vi "Delete remainig  reports at the begining.vi"() -> (0 "error out":errorcluster)   [LabVIEW 2023]
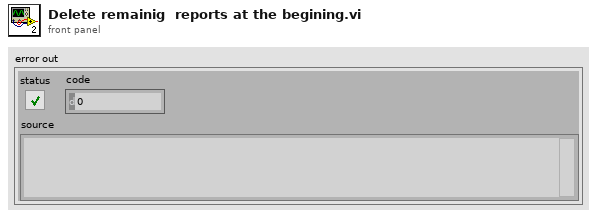
[diagram p1: front panel]
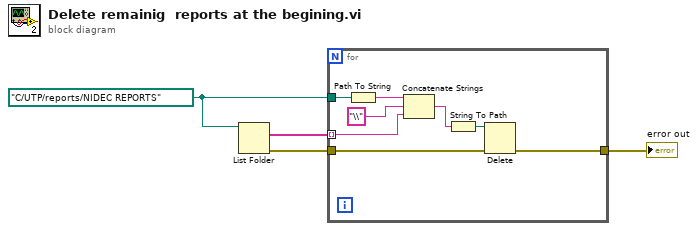
[diagram p0: block diagram]
diagram:
  w1 = path "C:/UTP/reports/NIDEC REPORTS" ("path")
  n1 = List Folder(path=w1) -> (filenames=w4:string[], error out=w3:errorcluster)  [unwired: 3 in, 2 out]
  n2 = for {
    tunnel: w4 -> [w6] mode=indexing
    tunnel: w3 -> [w12]
    tunnel: [w10] -> w2
    tunnel: w1 -> [w9]
    n3 = Path To String(path=w9) -> (string=w8:string)
    n4 = Concatenate Strings(w8, "\\" ("string"), w6) -> (w5:string)
    n5 = String To Path(string=w5) -> (path=w11:path)
    n6 = Delete(path (use dialog)=w11, error in=w12) -> (error out=w10:errorcluster)  [unwired: 3 in, 2 out]
  }
  "error out" <- w2
